vi "Clean_Up_Wrong_Calib_Filenames.vi"() -> ()   [LabVIEW 2011]
panel:
  out "Current raw data file":path
  out "x = y?":bool
  out "concatenated string":string
  out "Value":dbl=-999.0
  out "Recommended":string
  out "Original":string
  out "Checking":i32
  in  "Raw Data Folder":path=path "/EnFlo_Data/2012/EnFlo_Tunnel/Andrew_Burt/Calibrations"
  out "Array 2":dbl[](array[numeric]) format="%#.0f"
  out "Array":string[](array[string])
  in  "Calib Folder":path=path "/EnFlo_Data/2012/EnFlo_Tunnel/Andrew_Burt/Calibrations"
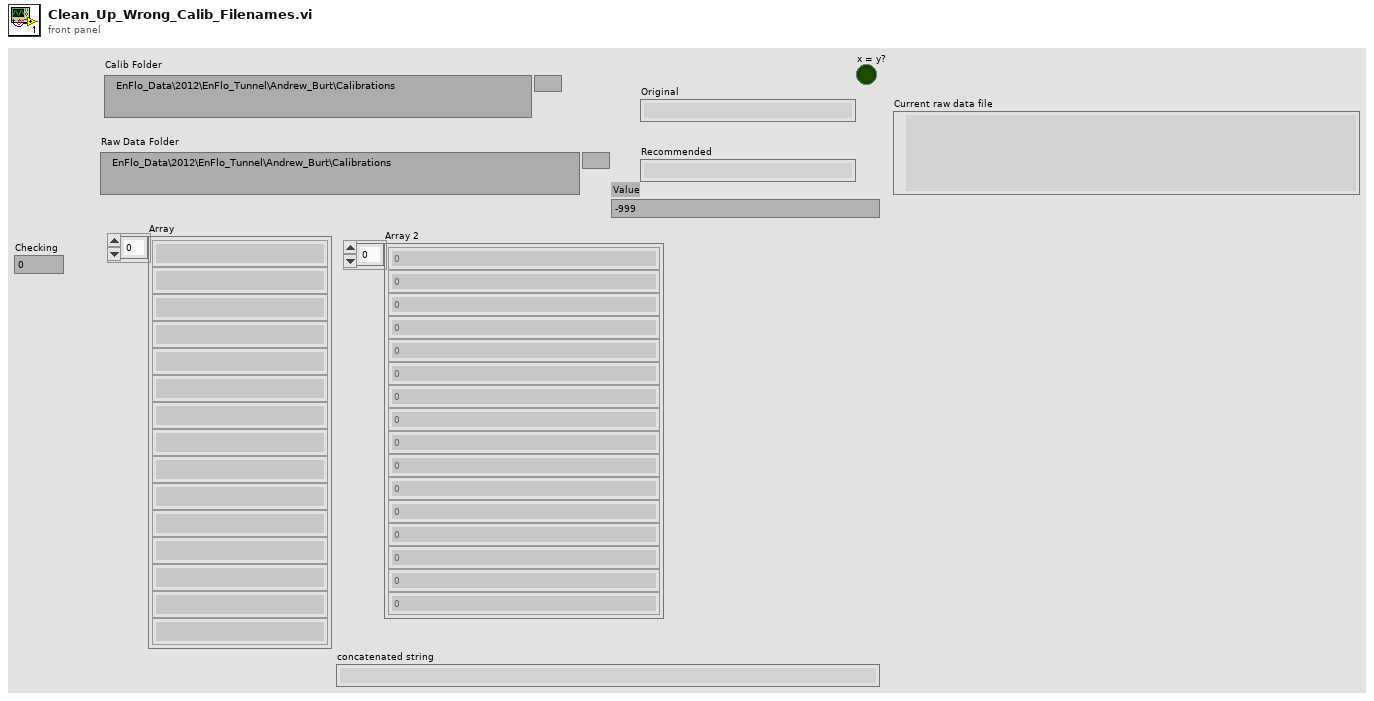
[diagram p1: front panel]
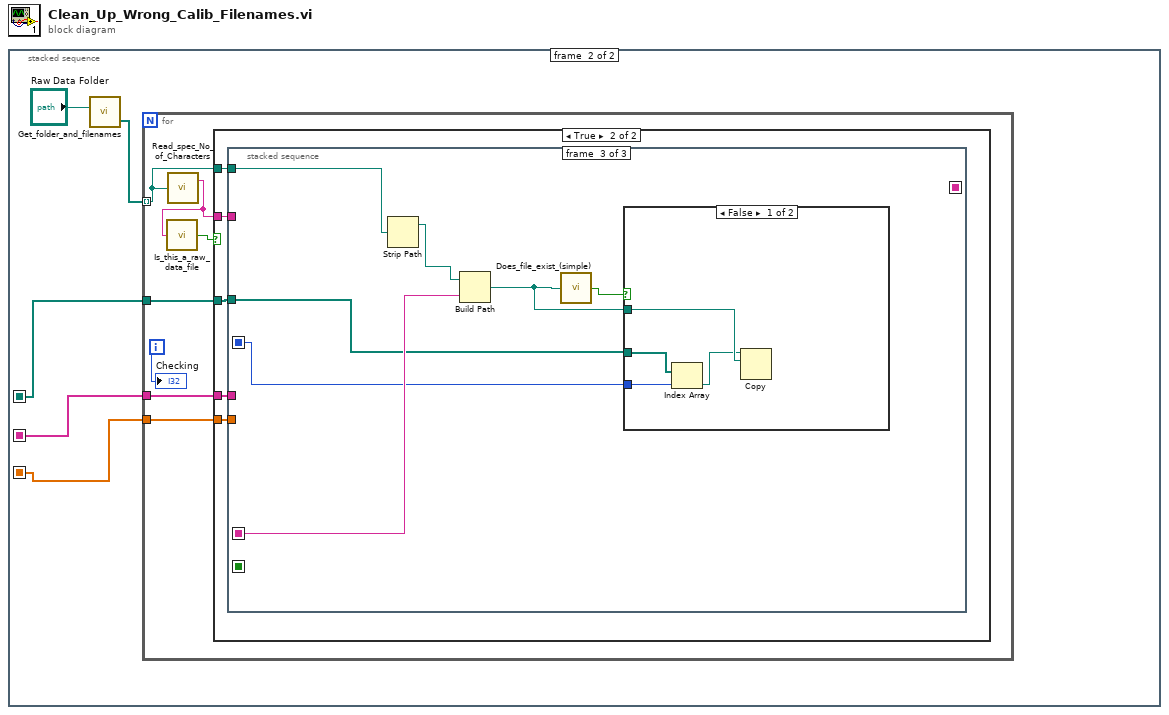
[diagram p0: block diagram]
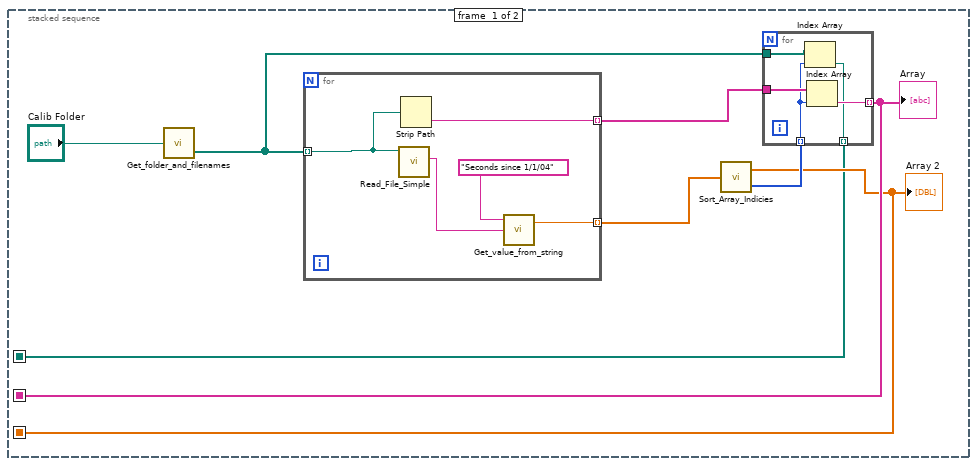
[diagram p2: hidden frame]
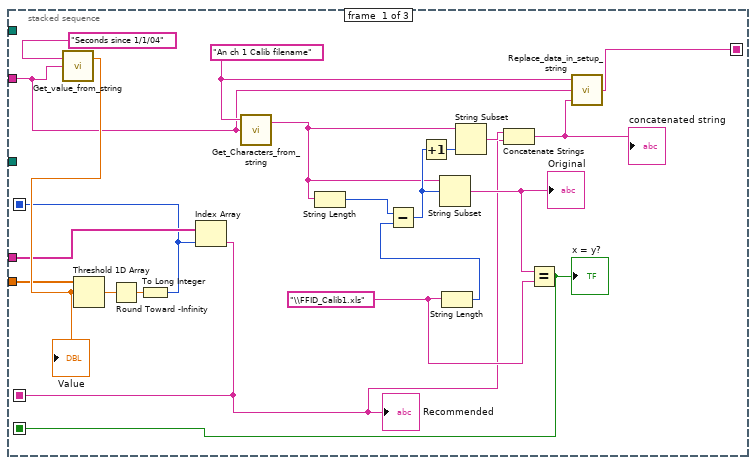
[diagram p4: hidden frame]
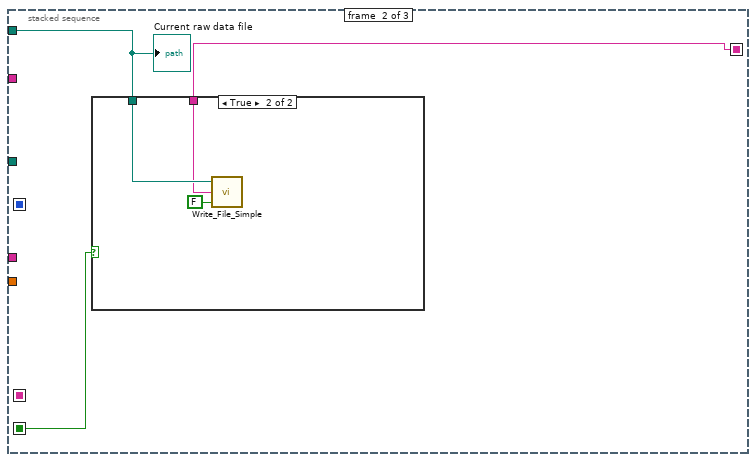
[diagram p5: hidden frame]
diagram:
  n1 = stacked-sequence {
    seq-local: [w4 _] -> [_ w20]
    seq-local: [w3 _] -> [_ w21]
    seq-local: [w1 _] -> [_ w19]
    frame #0 {
      n2 = call "Get_folder_and_filenames.vi"("file path (dialog if empty)"="Calib Folder") -> ("Files"=w2:path[])  [unwired: 1 out]
      n3 = for {
        tunnel: w2 -> [w18] mode=indexing
        tunnel: [w17] -> w5 mode=indexing
        tunnel: [w14] -> w7 mode=indexing
        n4 = call "Read_File_Simple.vi"("Filename"=w18) -> ("string"=w15:string)  [unwired: 4 in, 5 out]
        n5 = Strip Path(path=w18) -> (name=w17:string)  [unwired: 1 out]
        n6 = call "Get_value_from_string.vi"("Input string"=w15, "Variable name"="Seconds since 1/1/04") -> ("Value"=w14:dbl)  [unwired: 1 in, 1 out]
      }
      n7 = call "Sort_Array_Indicies.vi"("unsorted array"=w7) -> ("sorted array"=w3:dbl[], "Sort Index"=w6:i32[])
      "Array 2" <- w3
      n8 = for {
        tunnel: w6 -> [w11] mode=indexing
        tunnel: w5 -> [w13]
        tunnel: [w12] -> w4 mode=indexing
        tunnel: w2 -> [w10]
        tunnel: [w9] -> w1 mode=indexing
        n9 = Index Array(array=w10, index=w11) -> (element=w9:path)
        n10 = Index Array(array=w13, index=w11) -> (element=w12:string)
      }
      "Array" <- w4
    }
    frame #1 {
      n11 = call "Get_folder_and_filenames.vi"("file path (dialog if empty)"="Raw Data Folder") -> ("Files"=w22:path[])  [unwired: 1 out]
      n12 = for {
        tunnel: w22 -> [w29] mode=indexing
        tunnel: w21 -> [w26]
        tunnel: w20 -> [w25]
        tunnel: w19 -> [w24]
        i -> [w30]
        n13 = call "Read_spec_No_of_Characters.vi"("Filename"=w29) -> ("character string"=w27:string)  [unwired: 1 out]
        n14 = call "Is_this_a_raw_data_file.vi"("character string"=w27) -> ("Raw Dat File?"=w28:bool)  [unwired: 2 out]
        n15 = case shown="True" w28 {
          tunnel: w29 -> [_ w32]
          tunnel: w27 -> [_ w33]
          tunnel: w26 -> [_ w35]
          tunnel: w25 -> [_ w34]
          tunnel: w24 -> [_ w31]
          frame False {
          }
          frame True {
            n16 = stacked-sequence {
              seq-local: [w39 _ _] -> [_ w58 _]
              seq-local: [w38 _ _] -> [_ w57 _]
              seq-local: [w37 _ _] -> [_ _ w67]
              seq-local: [w36 _ _] -> [_ _ w63]
              tunnel: w35 -> [w54 _ _]
              tunnel: w34 -> [w51 _ _]
              tunnel: w33 -> [w45 _ _]
              tunnel: w32 -> [_ w59 w69]
              tunnel: w31 -> [_ _ w65]
              frame #0 {
                w47 = "\\FFID_Calib1.xls"
                w46 = "An ch 1 Calib filename" ("Variable name")
                n17 = call "Get_value_from_string.vi"("Input string"=w45, "Variable name"="Seconds since 1/1/04") -> ("Value"=w55:dbl)  [unwired: 1 in, 1 out]
                "Value" <- w55
                n18 = Threshold 1D Array(2:w55, 3:w54) -> (0:w53:dbl)  [unwired: 1 in]
                n19 = Round Toward -Infinity(1:w53) -> (0:w52:dbl)
                n20 = To Long Integer(number=w52) -> (32bit integer=w36:i32)
                n21 = Index Array(array=w51, index=w36) -> (element=w37:string)
                "Recommended" <- w37
                n22 = call "Get_Characters_from_string.vi"("Input string"=w45, "Variable name"=w46) -> ("Value"=w43:string)  [unwired: 1 in, 1 out]
                n23 = String Length(string=w43) -> (length=w50:i32)
                n24 = String Length(string=w47) -> (length=w49:i32)
                n25 = Subtract(x=w50, y=w49) -> (x-y=w44:i32)
                n26 = Increment(x=w44) -> (x+1=w40:i32)
                n27 = String Subset(string=w43, offset (0)=w44) -> (substring=w48:string)  [unwired: 1 in]
                "Original" <- w48
                n28 = String Subset(string=w43, length (rest)=w40) -> (substring=w42:string)  [unwired: 1 in]
                n29 = Concatenate Strings(w42, w37) -> (w41:string)
                "concatenated string" <- w41
                n30 = Equal?(x=w48, y=w47) -> (x = y?=w38:bool)
                "x = y?" <- w38
                n31 = call "Replace_data_in_setup_string.vi"("New data string"=w41, "Input string"=w45, "Variable name"=w46) -> ("Appended string"=w39:string)
              }
              frame #1 {
                n32 = case shown="True" w57 {
                  tunnel: w59 -> [_ w62]
                  tunnel: w58 -> [_ w61]
                  frame False {
                  }
                  frame True {
                    n33 = call "Write_File_Simple.vi"("append to file? (new file:F)"=FALSE, "character string"=w61, "file path"=w62) -> ()  [unwired: 2 out]
                  }
                }
                "Current raw data file" <- w59
              }
              frame #2 {
                n34 = Strip Path(path=w69) -> (stripped path=w68:path)  [unwired: 1 out]
                n35 = Build Path(base path=w68, name or relative path=w67) -> (appended path=w64:path)
                n36 = call "Does_file_exist_(simple).vi"("Pathname"=w64) -> ("exists?"=w66:bool)
                n37 = case shown="False" w66 {
                  tunnel: w65 -> [w71 _]
                  tunnel: w64 -> [w73 _]
                  tunnel: w63 -> [w72 _]
                  frame False {
                    n38 = Index Array(array=w71, index=w72) -> (element=w70:path)
                    n39 = Copy(10:w73, 11:w70) -> ()  [unwired: 3 in, 3 out]
                  }
                  frame True {
                  }
                }
              }
            }
          }
        }
        "Checking" <- w30
      }
    }
  }
